vi "Total cost of one paper.vi"(1 "Cost per day":dbl[](array[numeric]), 2 "Dates received":timestamp[](array[timestamp])) -> (0 "Total cost":dbl)   [LabVIEW 2015]
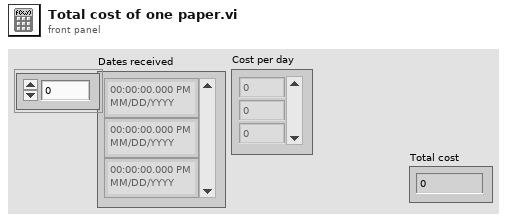
[diagram p1: front panel]
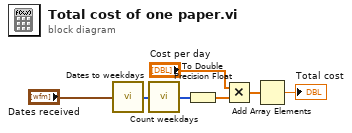
[diagram p0: block diagram]
diagram:
  n1 = call "Dates to weekdays.vi"("Dates"="Dates received") -> ("Weekdays"=w6:i32[])
  n2 = call "Count weekdays.vi"("Days"=w6) -> ("Day counts"=w3:i32[])
  n3 = To Double Precision Float(number=w3) -> (double precision float=w4:dbl[])
  n4 = Multiply(x="Cost per day", y=w4) -> (x*y=w2:dbl[])
  n5 = Add Array Elements(numeric array=w2) -> (sum=→"Total cost":dbl)
